vi "Init GFauswahl.vi"(8 "Fehler (Eingang, kein Fehler)":errorcluster, 10 "GF MFC3 (Eingang)":refnum<vi>, 11 "GF MFC2 (Eingang)":refnum<vi>) -> (0 "Fehler (Ausgang)":errorcluster, 2 "GF MFC3 (Ausgang)":refnum<vi>, 3 "GF MFC2 (Ausgang)":refnum<vi>)   [LabVIEW 2020, in "EPA 1065.lvlib" / "HovaCAL Interference verificaton.lvlib"]
uses:
  HovaCAL Interference verificaton.lvlib
  Seiten/System Einstellungen V2/System Einstellungen V2.lvlib
  Seiten/System Einstellungen V2/Aktion FGV Gasbottledefinition.ctl
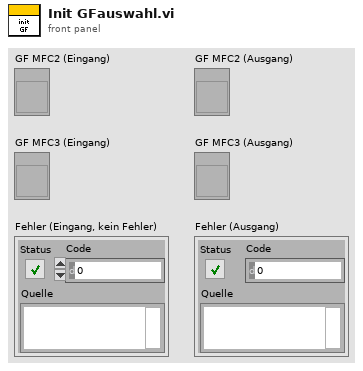
[diagram p1: front panel]
types:
  T1 = typedef "System Einstellungen V2.lvlib/Aktion FGV Gasbottledefinition.ctl" = enum16{"lesen", "schreiben", "löschen", "laden", "speichern", "exportieren", "importieren"}
  T2 = typedef "System Einstellungen V2.lvlib/Gasflasche gesamt.ctl" = cluster{"Gasflasche":T3, "Trägergas":T4, "Komponenten":T5[]}
  T3 = typedef "System Einstellungen V2.lvlib/Gasflasche.ctl" = cluster{"Gasname für die Auswahl":string, "Chargennummer":string, "Ablaufdatum":timestamp}
  T4 = typedef "System Einstellungen V2.lvlib/Traegergas.ctl" = string
  T5 = typedef "System Einstellungen V2.lvlib/Gasflaschenkomponente.ctl" = cluster{"Gasauswahl":string, "Konzentration IST":dbl, "Einheit":string, "Genauigkeit":dbl}
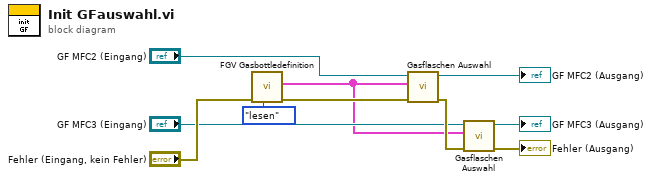
[diagram p0: block diagram]
diagram:
  n1 = call "FGV Gasbottledefinition.vi"("Aktion"=Aktion_FGV_Gasbottledefinition."lesen", "error in (no error)"="Fehler (Eingang, kein Fehler)") -> ("error out"=w7:errorcluster, "Gasflaschen Liste gesamt"=w4:T2[])  [unwired: 7 in, 1 out]
  n2 = call "Gasflaschen Auswahl.vi"("error in (no error)"=w7, "Gasflaschen Liste gesamt"=w4, "Ring (Eingang)"="GF MFC2 (Eingang)") -> ("error out"=w6:errorcluster, "Ring (Ausgang)"=→"GF MFC2 (Ausgang)":refnum<vi>)  [unwired: 6 in, 1 out]
  n3 = call "Gasflaschen Auswahl.vi"("error in (no error)"=w6, "Gasflaschen Liste gesamt"=w4, "Ring (Eingang)"="GF MFC3 (Eingang)") -> ("error out"=→"Fehler (Ausgang)":errorcluster, "Ring (Ausgang)"=→"GF MFC3 (Ausgang)":refnum<vi>)  [unwired: 6 in, 1 out]
